vi "ConfigDOClock.vi"(0 "object in":refnum<class "AD2_SDK.lvclass">, 1 "DO Trigger":T2, 2 "ClockSettings":T1(array[cluster]), 5 "error in (no error)":errorcluster) -> (14 "object out":refnum<class "AD2_SDK.lvclass">, 19 "error out":errorcluster)   [LabVIEW 2024, in "AD2_SDK.lvclass"]
uses:
  AD2_SDK.lvclass
  AD2_DO_SDK_class/DOTrigger.ctl
  AD2_WFG_SDK_class/AD2TriggerSources.ctl
  AD2_SDK.lvclass/AD2_SDK.ctl
  AD2_DO_SDK_class/AD2_DO_SDK.lvclass
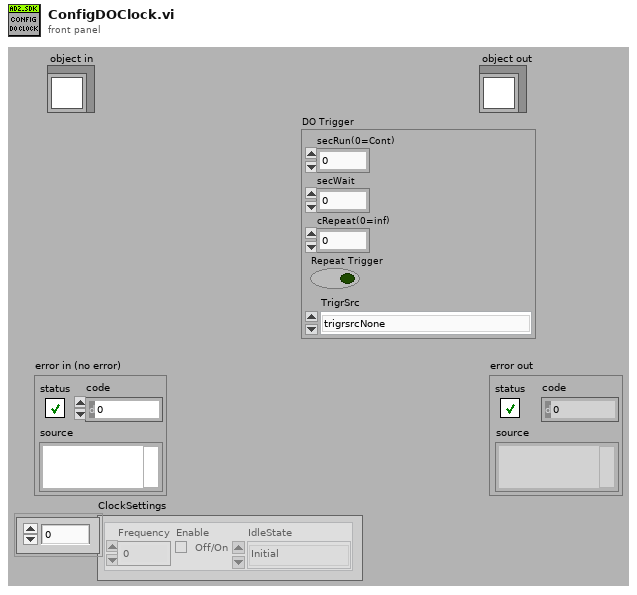
[diagram p1: front panel]
types:
  T1 = cluster{"Frequency":dbl, "Enable":bool, "IdleState":enum16{"Initial", "Low", "High", "Z"}}[]
  T2 = typedef "AD2_DO_SDK.lvclass/DOTrigger.ctl" = cluster{"secRun(0=Cont)":dbl, "secWait":dbl, "cRepeat(0=inf)":i32, "Repeat Trigger":bool, "TrigrSrc":T3}
  T3 = typedef "AD2_SDK.lvclass/AD2TriggerSources.ctl" = enum8{"trigrsrcNone", "trigsrcPC", "trigsrcDetectorAnalogIn", "trigsrcDetectorDigitalIn", "trigsrcAnalogIn", "trigsrcDigitalIn", "trigsrcDigitalOut", "trigsrcAnalogOut1", "trigsrcAnalogOut2", "trigsrcAnalogOut3", "trigsrcAnalogOut4", "trigsrcExternal1", "trigsrcExternal2", "trigsrcExternal3", "trigsrcExternal4", ""}
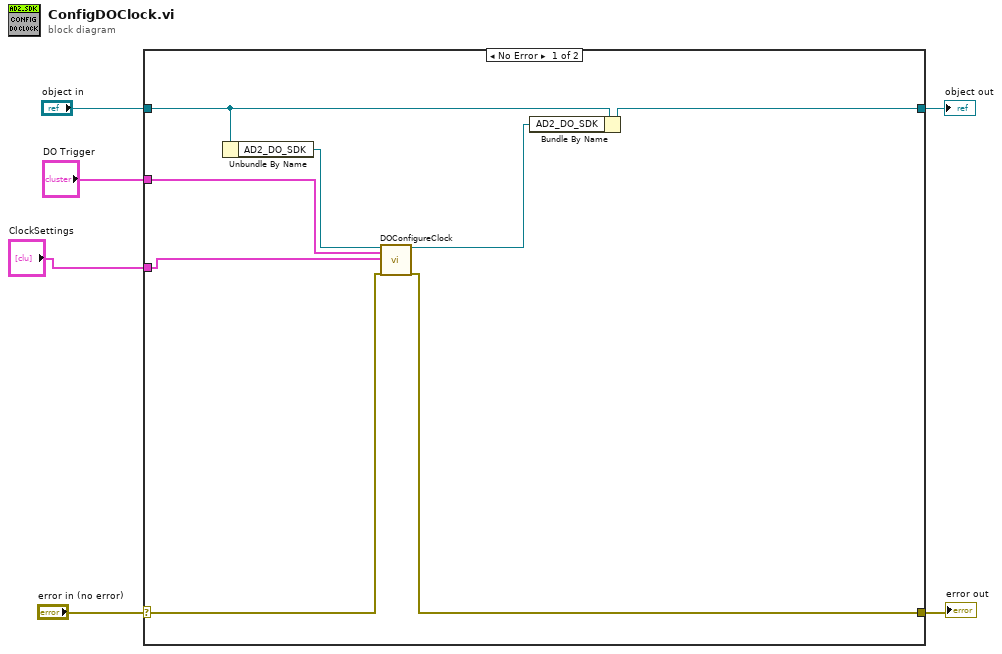
[diagram p0: block diagram]
diagram:
  n1 = case shown="No Error" "error in (no error)" {
    selector: "error in (no error)" -> [w10 w16]
    tunnel: [w9 w16] -> w5
    tunnel: [w12 w15] -> w3
    tunnel: "object in" -> [w14 w15]
    tunnel: "DO Trigger" -> [w8 _]
    tunnel: "ClockSettings" -> [w7 _]
    frame No Error {
      n2 = Unbundle By Name(w14) -> ("AD2_DO_SDK"=w13:refnum<class "AD2_DO_SDK.lvclass">)
      n3 = call-dynamic "DOConfigureClock.vi"("object in"=w13, "DO Trigger"=w8, "ClockSettings"=w7, "error in (no error)"=w10) -> ("object out"=w11:refnum<class "AD2_DO_SDK.lvclass">, "error out"=w9:errorcluster)  [unwired: 14 in]
      n4 = Bundle By Name(cluster=w14, "AD2_DO_SDK"=w11) -> (w12:refnum<class "AD2_SDK.lvclass">)
    }
    frame Error {
    }
  }
  "error out" <- w5
  "object out" <- w3
